vi "Configure AI Buffer.vi"(8 "error in (no error)":errorcluster, 11 "Refnum in":refnum<k21>) -> (0 "error out":errorcluster, 3 "Refnum out":refnum<k21>)   [LabVIEW 2014, in "DAQmx Module Runtime.lvclass"]
uses:
  DAQmx Module Runtime.lvclass
  <resource>/objmgr/daqmx.rc
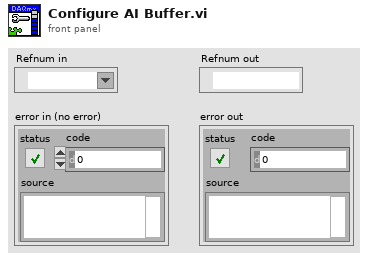
[diagram p1: front panel]
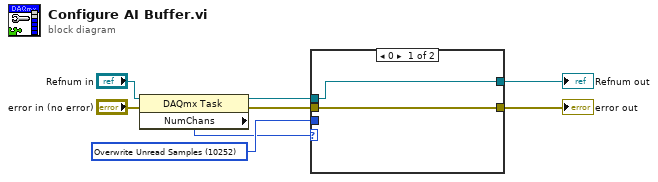
[diagram p0: block diagram]
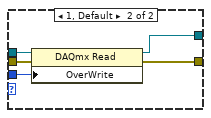
[diagram p2: hidden frame]
diagram:
  w6 = 10252 items=["Overwrite Unread Samples"=10252, "Do Not Overwrite Unread Samples"=10159] ("OverWrite")
  n1 = property class="DAQmx Task"(reference="Refnum in", error in="error in (no error)") -> (reference out=w4:refnum<k21>, error out=w2:errorcluster, "NumChans"=w1:u32)
  n2 = case shown="0" w1 {
    tunnel: [w10 w15] -> w8
    tunnel: [w9 w14] -> w7
    tunnel: w6 -> [_ w13]
    tunnel: w4 -> [w10 w12]
    tunnel: w2 -> [w9 w11]
    frame 0 {
    }
    frame 1, Default {
      n3 = property class="DAQmx Read"(reference=w12, error in=w11, "OverWrite"=w13) -> (reference out=w15:refnum<k21>, error out=w14:errorcluster)
    }
  }
  "Refnum out" <- w8
  "error out" <- w7
